vi "OM_FromLabVIEW.vi"(8 "error in (no error)":errorcluster, 11 "syslogs in":refnum<class "syslogs.lvclass">) -> (0 "error out":errorcluster, 2 "DbRow":variant, 3 "syslogs out":refnum<class "syslogs.lvclass">)   [LabVIEW 2020, in "ORM_Examples.lvlib" / "syslogs.lvclass"]
uses:
  syslogs.lvclass
  syslogs.lvclass/syslogs.ctl
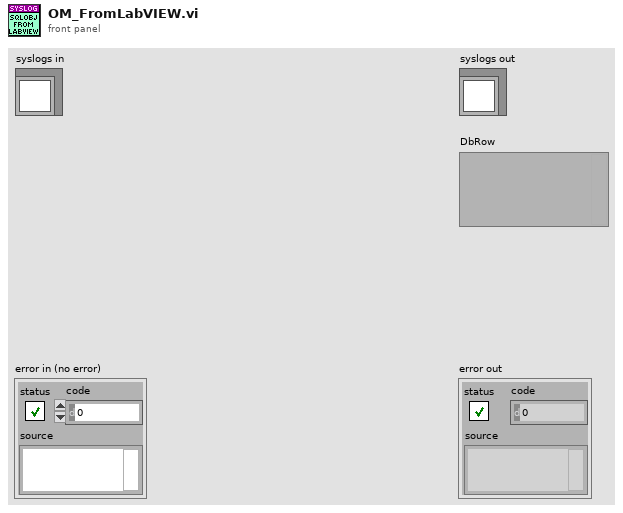
[diagram p1: front panel]
types:
  T1 = typedef "type.ctl" = string
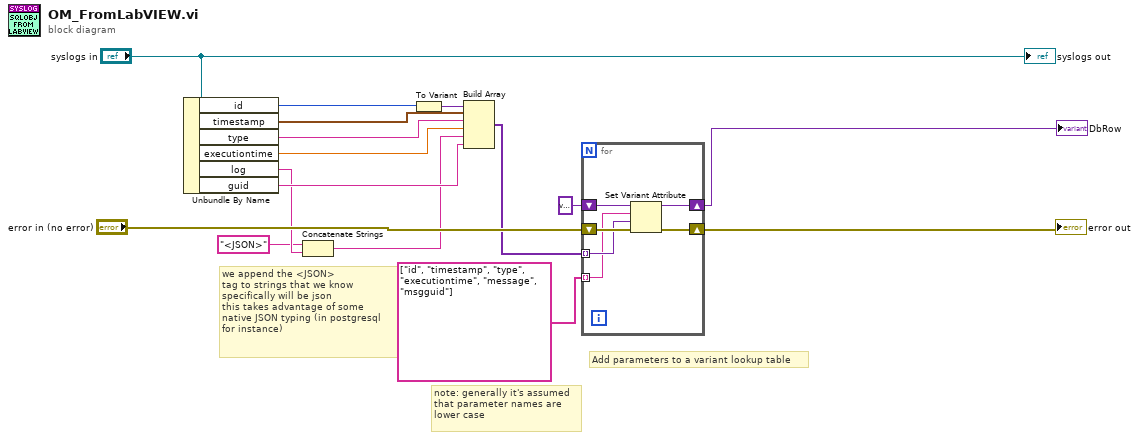
[diagram p0: block diagram]
diagram:
  # "we append the <JSON>\ntag to strings that we know\nspecifically will be json\nthis takes advantage of some\nnative JSON typing (in postgresql\nfor instance)"
  # "note: generally it's assumed\nthat parameter names are \nlower case"
  # "Add parameters to a variant lookup table"
  n1 = Unbundle By Name("syslogs in") -> ("id"=w15:i32, "timestamp"=w13:timestamp, "type"=w12:T1, "executiontime"=w11:dbl, "log"=w3:string, "guid"=w10:string)
  n2 = Concatenate Strings("<JSON>" ("string"), w3) -> (w2:string)
  n3 = To Variant(anything=w15) -> (Variant=w14:variant)
  n4 = Build Array(w14, w13, w12, w11, w2, w10) -> (w5:variant[])
  n5 = for {
    shift-right: [w21] -> w8
    shift-left: "error in (no error)" -> [w22]
    shift-right: [w20] -> w7
    shift-left: variant -> [w19]
    tunnel: w5 -> [w18] mode=indexing
    tunnel: string[] ["id", "timestamp", "type", "executiontime", "message", "msgguid"] -> [w17] mode=indexing
    n6 = Set Variant Attribute(Variant=w19, name=w17, value=w18, error in=w22) -> (Variant out=w20:variant, error out=w21:errorcluster)  [unwired: 1 out]
  }
  "error out" <- w8
  "DbRow" <- w7
  "syslogs out" <- "syslogs in"
